vi "行列索引2D数组(CSG).vi"(8 "error in (no error)":errorcluster caption="错误输入（无错误）", 10 "索引":cluster{"行":i32, "列":i32}[](array[cluster]), 11 "输入数组":csg[][](array[numeric])) -> (0 "error out":errorcluster caption="错误输出", 3 "元素":csg[](array[numeric]))   [LabVIEW 2012]
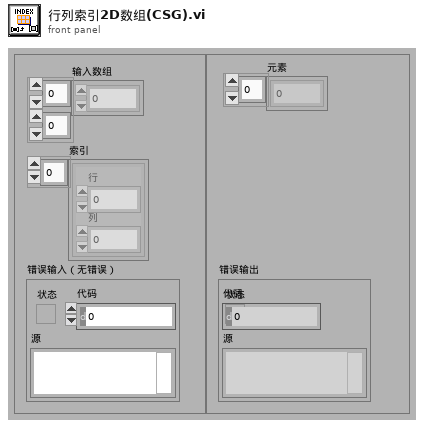
[diagram p1: front panel]
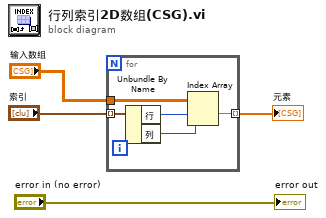
[diagram p0: block diagram]
diagram:
  n1 = for {
    tunnel: "索引" -> [w7] mode=indexing
    tunnel: "输入数组" -> [w9]
    tunnel: [w8] -> w1 mode=indexing
    n2 = Unbundle By Name(w7) -> ("行"=w6:i32, "列"=w5:i32)
    n3 = Index Array(array=w9, index (row)=w6, index (col)=w5) -> (element=w8:csg)
  }
  "元素" <- w1
  "error out" <- "error in (no error)"
